vi "Display n or dt.vi"(8 "error in (no error)":errorcluster, 10 "X Axis":T1=enum."Samples" caption="Enum", 11 "Input Waveforms":waveform(dbl)[](array[waveform])) -> (0 "error out":errorcluster, 3 "Output Waveforms":waveform(dbl)[](array[waveform]))   [LabVIEW 2019, in "Instrument UI.Lockin.lvclass"]
uses:
  Instrument UI.Lockin.lvclass
  Typedefs/X Axis-Enum.ctl
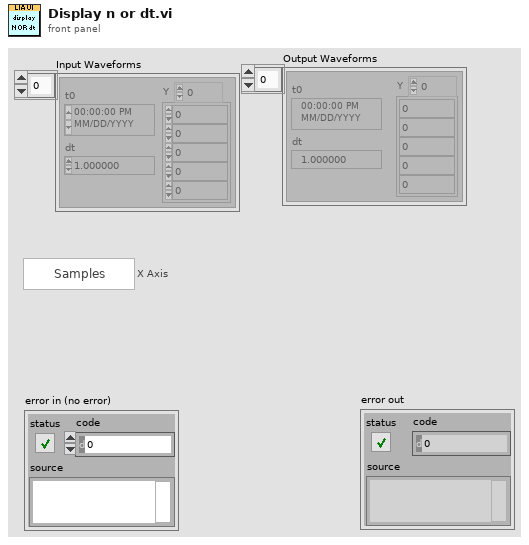
[diagram p1: front panel]
types:
  T1 = typedef "Instrument UI.Lockin.lvclass/X Axis-Enum.ctl" = enum16{"Time", "Samples"}
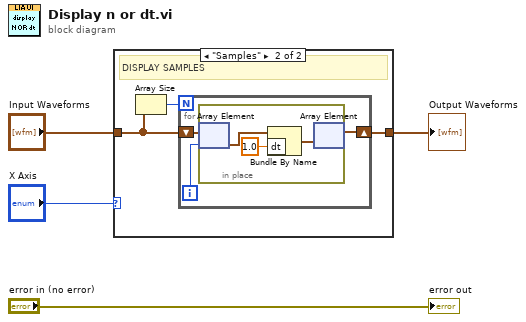
[diagram p0: block diagram]
diagram:
  n1 = case shown="\"Samples\"" "X Axis" {
    tunnel: [w5 w8] -> w4
    tunnel: "Input Waveforms" -> [w5 w6]
    frame "Time", Default {
      # "Display Time"
    }
    frame "Samples" {
      # "DISPLAY SAMPLES"
      n2 = Array Size(array=w6) -> (size(s)=w7:i32)
      n3 = for {
        N: w7 -> [_]
        shift-right: [w9] -> w8
        shift-left: w6 -> [w10]
        i -> [w11]
        n4 = in-place {
          n5 = in-place-array #1(w10, w11) -> (w12:waveform(dbl))
          n6 = Bundle By Name(cluster=w12, "dt"=1.0) -> (w13:waveform(dbl))
          n7 = in-place-array #1(w13) -> (w9:waveform(dbl)[])  [unwired: 1 out]
        }
      }
    }
  }
  "Output Waveforms" <- w4
  "error out" <- "error in (no error)"
